vi "Get Meta Parameters.vi"(8 "error in":errorcluster) -> (0 "error out":errorcluster, 3 "measurement_parameters":T1)   [LabVIEW 2020, in "LoadRegulation.lvlib" / "MeasurementService_Template.lvclass"]
uses:
  MeasurementService_Template.lvclass
  RPC Messages/Measurement_v1_MeasurementParameters/Measurement_v1_MeasurementParameters_Data.ctl
  RPC Messages/Measurement_v1_ConfigurationParameter/Measurement_v1_ConfigurationParameter_Data.ctl
  RPC Messages/Measurement_v1_OutputParameter/Measurement_v1_OutputParameter_Data.ctl
  Measurement Configuration.ctl
  Measurement Results.ctl
  LoadRegulation.lvlib
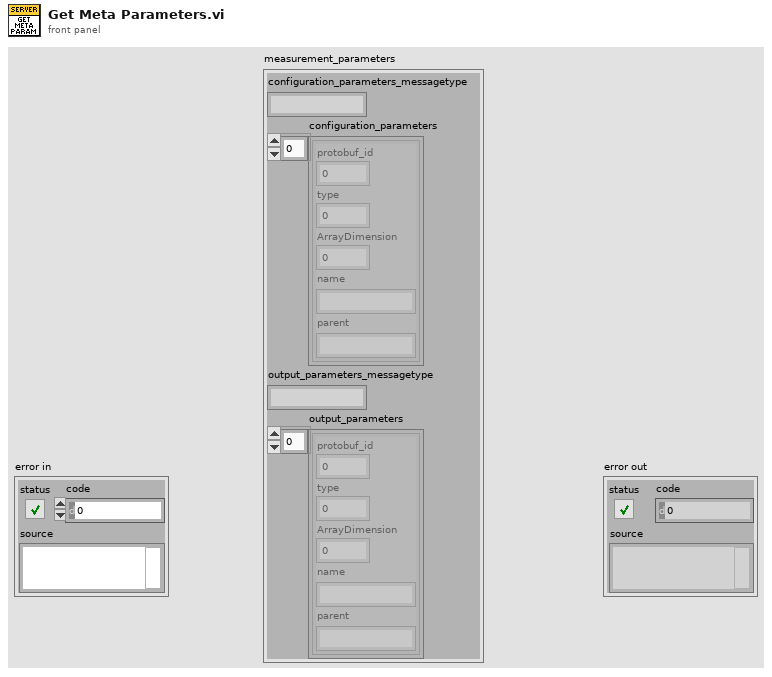
[diagram p1: front panel]
types:
  T1 = typedef "LoadRegulation.lvlib/MeasurementService_Template.lvclass/Measurement_v1_MeasurementParameters_Data.ctl" = cluster{"configuration_parameters_messagetype":string, "configuration_parameters":T2[], "output_parameters_messagetype":string, "output_parameters":T3[]}
  T2 = typedef "LoadRegulation.lvlib/MeasurementService_Template.lvclass/Measurement_v1_ConfigurationParameter_Data.ctl" = cluster{"protobuf_id":i32, "type":i32, "ArrayDimension":i32, "name":string, "parent":string}
  T3 = typedef "LoadRegulation.lvlib/MeasurementService_Template.lvclass/Measurement_v1_OutputParameter_Data.ctl" = cluster{"protobuf_id":i32, "type":i32, "ArrayDimension":i32, "name":string, "parent":string}
  T4 = typedef "LoadRegulation.lvlib/Measurement Results.ctl" = cluster{"Load Regulation (%)":dbl, "Load Regulation (mV/mA)":dbl, "Test Results.Load Current in A":dbl[], "Output Voltage in V":dbl[]}
  T5 = typedef "LoadRegulation.lvlib/Measurement Configuration.ctl" = cluster{"Input Voltage in V":dbl, "Nominal Output Voltage in V":dbl, "Start":dbl, "Stop":dbl, "Step":dbl, "Input SMU":string, "Load SMU":string, "Input DMM":string, "Load DMM":string}
  T6 = cluster{"protobuf_id":i32, "type":i32, "ArrayDimension":i32, "name":string, "parent":string}[]
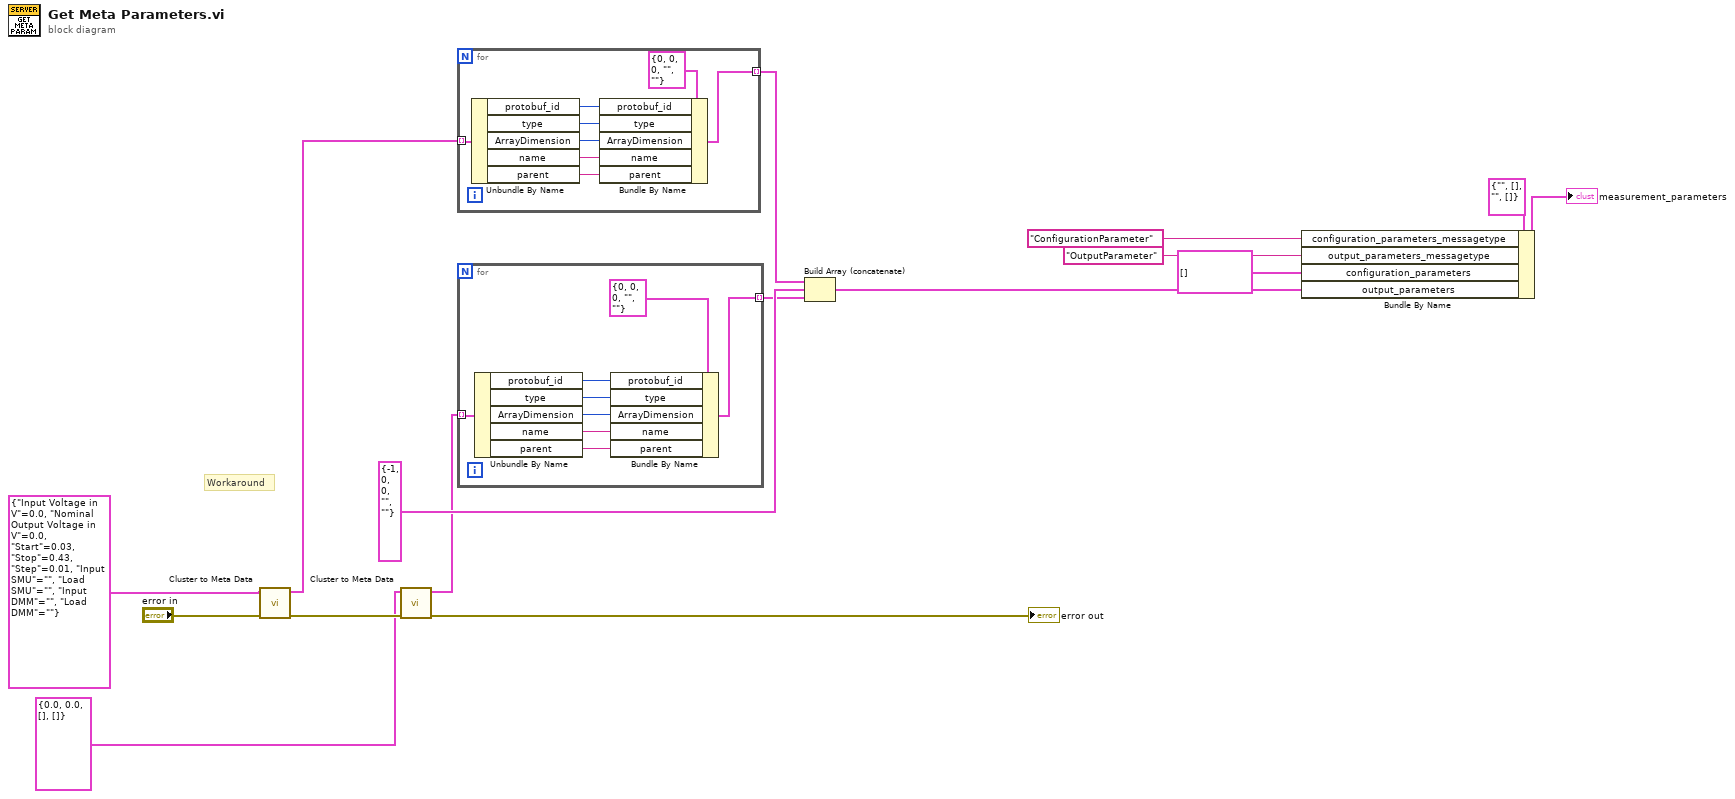
[diagram p0: block diagram]
diagram:
  # "Workaround"
  n1 = call "Cluster to Meta Data.vi"("error in"="error in", "Configuration Cluster"=T5 {"Input Voltage in V"=0.0, "Nominal Output Voltage in V"=0.0, "Start"=0.03, "Stop"=0.43, "Step"=0.01, "Input SMU"="", "Load SMU"="", "Input DMM"="", "Load DMM"=""} ("Measurement Configuration")) -> ("error out"=w7:errorcluster, "configuration_parameters"=w4:T6)  [unwired: 8 in]
  n2 = call "Cluster to Meta Data.vi"("error in"=w7, "Configuration Cluster"=T4 {"Load Regulation (%)"=0.0, "Load Regulation (mV/mA)"=0.0, "Test Results.Load Current in A"=[], "Output Voltage in V"=[]} ("Measurement Results")) -> ("error out"=→"error out":errorcluster, "configuration_parameters"=w2:T6)  [unwired: 8 in]
  n3 = for {
    tunnel: w4 -> [w24] mode=indexing
    tunnel: [w17] -> w3 mode=indexing
    n4 = Unbundle By Name(w24) -> ("protobuf_id"=w22:i32, "type"=w21:i32, "ArrayDimension"=w20:i32, "name"=w19:string, "parent"=w18:string)
    n5 = Bundle By Name(cluster=T2 {"protobuf_id"=0, "type"=0, "ArrayDimension"=0, "name"="", "parent"=""} ("Measurement_v1_ConfigurationParameter_Data"), "protobuf_id"=w22, "type"=w21, "ArrayDimension"=w20, "name"=w19, "parent"=w18) -> (w17:T2)
  }
  n6 = for {
    tunnel: w2 -> [w32] mode=indexing
    tunnel: [w26] -> w1 mode=indexing
    n7 = Unbundle By Name(w32) -> ("protobuf_id"=w31:i32, "type"=w30:i32, "ArrayDimension"=w29:i32, "name"=w28:string, "parent"=w27:string)
    n8 = Bundle By Name(cluster=T3 {"protobuf_id"=0, "type"=0, "ArrayDimension"=0, "name"="", "parent"=""} ("Measurement_v1_OutputParameter_Data"), "protobuf_id"=w31, "type"=w30, "ArrayDimension"=w29, "name"=w28, "parent"=w27) -> (w26:T3)
  }
  n9 = Build Array (concatenate)(w3, T2 {"protobuf_id"=-1, "type"=0, "ArrayDimension"=0, "name"="", "parent"=""} ("Measurement_v1_ConfigurationParameter_Data"), w1) -> (w8:T3[])
  n10 = Bundle By Name(cluster=T1 {"configuration_parameters_messagetype"="", "configuration_parameters"=[], "output_parameters_messagetype"="", "output_parameters"=[]} ("measurement_parameters"), "configuration_parameters_messagetype"="ConfigurationParameter", "output_parameters_messagetype"="OutputParameter" ("configuration_parameters_messagetype"), "configuration_parameters"=T2[] [], "output_parameters"=w8) -> (→"measurement_parameters":T1)
